vi "Init.vi"(8 "error in (no error)":errorcluster, 9 "Type":i32, 10 "ID":string, 11 "Effect in":refnum<class "Effect.lvclass">) -> (0 "error out":errorcluster, 3 "Effect out":refnum<class "Effect.lvclass">)   [LabVIEW 2019, in "Effect.lvclass"]
uses:
  Effect.lvclass
  Libraries/Audio Processing/Value Cluster.ctl
  Libraries/Audio Processing/Value Properties.ctl
  Effect.lvclass/Effect.ctl
  Libraries/Messaging/Messaging.lvlib
  Libraries/Audio Processing/Audio Processing.lvlib
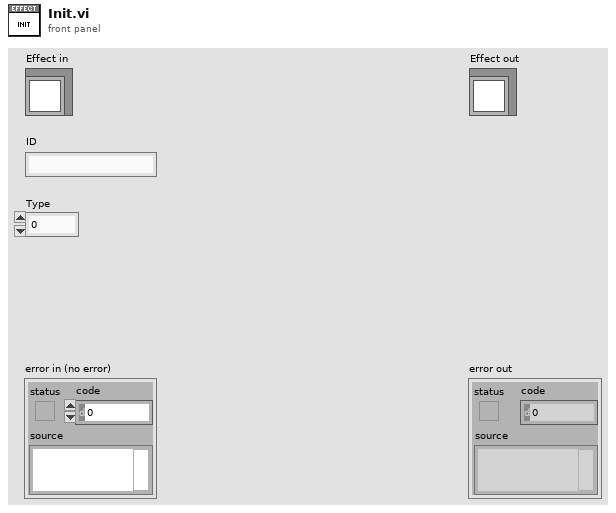
[diagram p1: front panel]
types:
  T1 = typedef "Audio Processing.lvlib/Value Cluster.ctl" = cluster{"Value":dbl, "Limits":T2}
  T2 = typedef "Audio Processing.lvlib/Value Properties.ctl" = cluster{"Lower":dbl, "Upper":dbl}
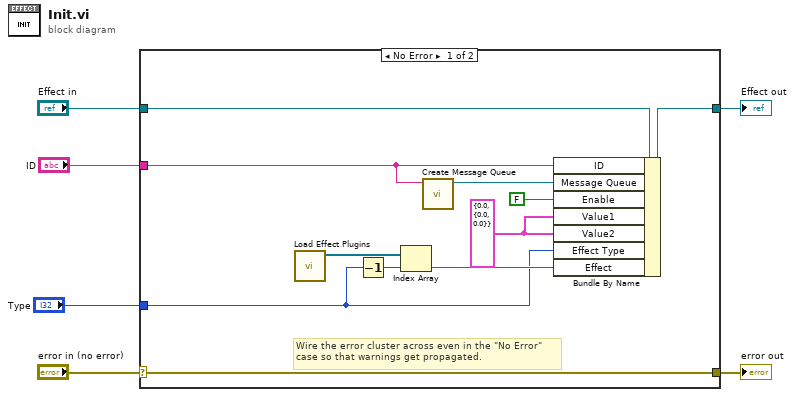
[diagram p0: block diagram]
diagram:
  n1 = case shown="No Error" "error in (no error)" {
    selector: "error in (no error)" -> [w17 w19]
    tunnel: [w17 w19] -> w5
    tunnel: [w16 w18] -> w3
    tunnel: "Effect in" -> [w15 w18]
    tunnel: "ID" -> [w13 _]
    tunnel: "Type" -> [w8 _]
    frame No Error {
      w11 = T1 {"Value"=0.0, "Limits"={"Lower"=0.0, "Upper"=0.0}} ("Value1")
      # "Wire the error cluster across even in the \"No Error\"\ncase so that warnings get propagated."
      n2 = call "Load Effect Plugins.vi"() -> ("Effect Plugins"=w10:refnum<class "Effect Interface.lvclass">[])  [unwired: 11 in]
      n3 = Decrement(x=w8) -> (x-1=w7:i32)
      n4 = Index Array(array=w10, index=w7) -> (element=w9:refnum<class "Effect Interface.lvclass">)
      n5 = call "Create Message Queue.vi"("Queue Name"=w13) -> ("queue out"=w12:refnum<queue>)  [unwired: 9 in, 1 out]
      n6 = Bundle By Name(cluster=w15, "ID"=w13, "Message Queue"=w12, "Enable"=FALSE ("Enabled"), "Value1"=w11, "Value2"=w11, "Effect Type"=w8, "Effect"=w9) -> (w16:refnum<class "Effect.lvclass">)
    }
    frame Error {
    }
  }
  "error out" <- w5
  "Effect out" <- w3
